vi "Voice Init.vi"(8 "Error In":errorcluster, 11 "Text":refnum<vi>) -> (0 "Error Out":errorcluster, 2 "Event Callback":refnum<k27>, 3 "Reference":refnum<k24>)   [LabVIEW 2018]
uses:
  System.Speech
panel:
  in  "CMD List":string[](array[string])
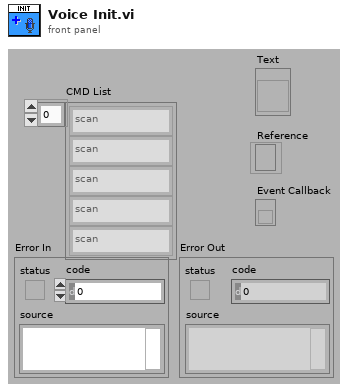
[diagram p1: front panel]
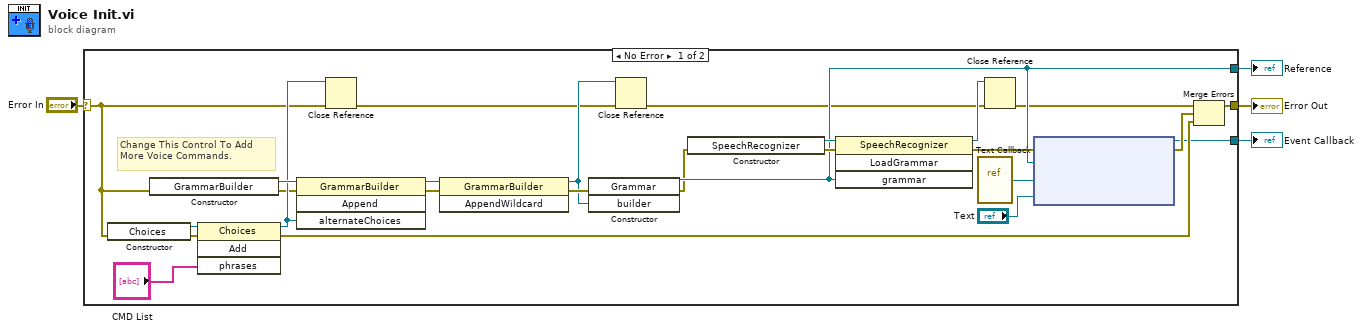
[diagram p0: block diagram]
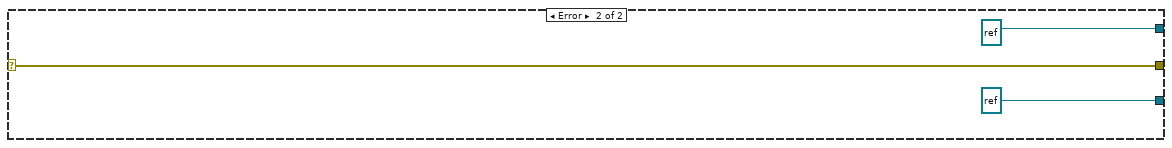
[diagram p2: hidden frame]
diagram:
  n1 = case shown="No Error" "Error In" {
    selector: "Error In" -> [w13 w33]
    tunnel: [w7 refnum<k27> refnum ("Event Callback")] -> w3
    tunnel: [w16 refnum<k24> refnum ("new reference")] -> w2
    tunnel: [w11 w33] -> w1
    frame No Error {
      # "Change This Control To Add More Voice Commands."
      n2 = constructor class="Choices"(error in=w13) -> (reference out=w22:refnum<k24>, error out=w24:errorcluster)  [unwired: 2 in, 1 out]
      n3 = constructor class="GrammarBuilder"(error in=w13) -> (reference out=w20:refnum<k24>, error out=w9:errorcluster)  [unwired: 2 in, 1 out]
      n4 = invoke class="Choices" method="Add"(reference=w22, error in=w24, "phrases"="CMD List") -> (reference out=w19:refnum<k24>, error out=w8:errorcluster)  [unwired: 1 in, 2 out]
      n5 = invoke class="GrammarBuilder" method="Append"(reference=w20, error in=w9, "alternateChoices"=w19) -> (reference out=w23:refnum<k24>, error out=w21:errorcluster)  [unwired: 1 in, 2 out]
      n6 = Close Reference(reference=w19, error in (no error)=w13) -> (error out=w14:errorcluster)
      n7 = invoke class="GrammarBuilder" method="AppendWildcard"(reference=w23, error in=w21) -> (reference out=w18:refnum<k24>, error out=w27:errorcluster)  [unwired: 1 in, 1 out]
      n8 = constructor class="Grammar"(error in=w27, "builder"=w18) -> (reference out=w16:refnum<k24>, error out=w6:errorcluster)  [unwired: 2 in, 2 out]
      n9 = Close Reference(reference=w18, error in (no error)=w14) -> (error out=w15:errorcluster)
      n10 = constructor class="SpeechRecognizer"(error in=w6) -> (reference out=w29:refnum<k24>, error out=w30:errorcluster)  [unwired: 2 in, 1 out]
      n11 = invoke class="SpeechRecognizer" method="LoadGrammar"(reference=w29, error in=w30, "grammar"=w16) -> (reference out=w17:refnum<k24>, error out=w28:errorcluster)  [unwired: 1 in, 2 out]
      n12 = vi-ref "Text Callback.vi"() -> (w25:refnum<vi>)
      n13 = Close Reference(reference=w17, error in (no error)=w15) -> (error out=w12:errorcluster)
      n14 = node(w28, w16, w25, "Text") -> (w7:refnum<k27>, w10:errorcluster)  [unwired: 1 in]
      n15 = Merge Errors(w12, w10, w8) -> (w11:errorcluster)
    }
    frame Error {
    }
  }
  "Error Out" <- w1
  "Event Callback" <- w3
  "Reference" <- w2
